vi "fileAsynchronousWrite.vi"(1 "line":string) -> ()   [LabVIEW 2017]
uses:
  globalUtilities.vi
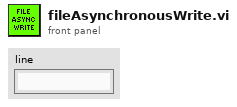
[diagram p1: front panel]
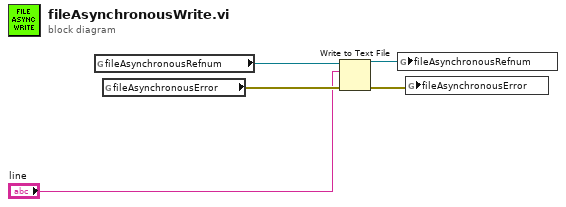
[diagram p0: block diagram]
diagram:
  n1 = global read "globalUtilities.vi" "fileAsynchronousRefnum"() -> (w5:refnum<file>)
  n2 = global read "globalUtilities.vi" "fileAsynchronousError"() -> (w4:errorcluster)
  n3 = Write to Text File(file (use dialog)=w5, text="line", error in=w4) -> (refnum out=w2:refnum<file>, error out=w1:errorcluster)  [unwired: 1 in, 1 out]
  n4 = global write "globalUtilities.vi" "fileAsynchronousRefnum"(w2) -> ()
  n5 = global write "globalUtilities.vi" "fileAsynchronousError"(w1) -> ()
